vi "BRig_dataCurrent_FreeReward_c.vi"() -> (2 "output_FreeReward_c":i32)   [LabVIEW 2014]
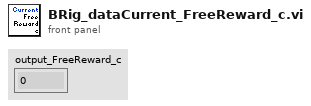
[diagram p1: front panel]
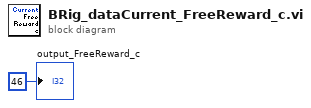
[diagram p0: block diagram]
diagram:
  "output_FreeReward_c" <- 46 ("output_iBlock")
